vi "SSC DAQmx Disable Start Trigger.vi"(0 "DAQmx SSC in":T1[](array[typedef]), 11 "error in":errorcluster) -> (4 "DAQmx SSC out":T1[](array[typedef]), 15 "error out":errorcluster)   [LabVIEW 2020]
doc: "Configures the task to start acquiring or generating samples immediately upon starting the task."
uses:
  Pin Map/SSC DAQmx.ctl
  <vilib>/DAQmx/configure/trigger.llb/DAQmx Start Trigger (None).vi
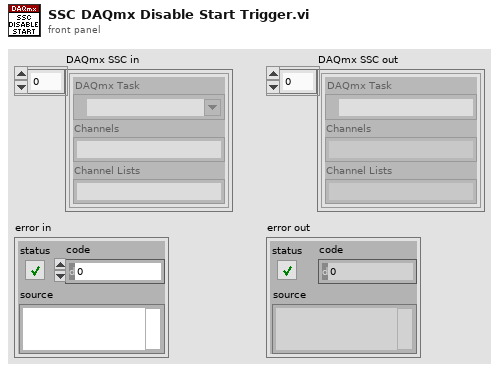
[diagram p1: front panel]
types:
  T1 = typedef "SSC DAQmx.ctl" = cluster{"DAQmx Task ":refnum<k21>, "Channels":string, "Channel Lists":string}
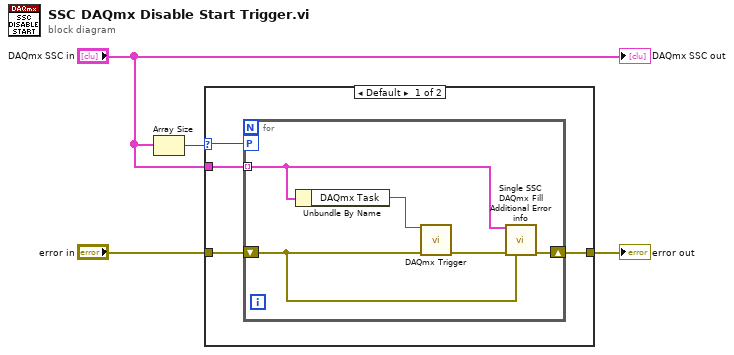
[diagram p0: block diagram]
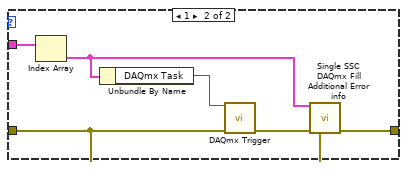
[diagram p2: hidden frame]
diagram:
  n1 = Array Size(array="DAQmx SSC in") -> (size(s)=w2:i32)
  n2 = case shown="Default" w2 {
    selector: w2 -> [w6 _]
    tunnel: [w8 w19] -> w4
    tunnel: "error in" -> [w7 w18]
    tunnel: "DAQmx SSC in" -> [w5 w17]
    frame Default {
      n3 = for {
        tunnel: w5 -> [w12] mode=indexing
        workers-P: w6 -> [_]
        shift-right: [w13] -> w8
        shift-left: w7 -> [w11]
        n4 = Unbundle By Name(w12) -> ("DAQmx Task"=w9:refnum<k21>)
        n5 = call-poly <vilib>:"DAQmx Trigger.vi"("task/channels in"=w9, "error in"=w11) -> ("error out"=w10:errorcluster)  [unwired: 12 in, 1 out]
        n6 = call "Single SSC DAQmx Fill Additional Error info.vi"("DAQmx SSC in"=w12, "error in"=w10, "previous error in"=w11) -> ("error out"=w13:errorcluster)  [unwired: 12 in]
      }
    }
    frame 1 {
      n7 = Index Array(array=w17) -> (element=w14:T1)  [unwired: 1 in]
      n8 = Unbundle By Name(w14) -> ("DAQmx Task"=w15:refnum<k21>)
      n9 = call-poly <vilib>:"DAQmx Trigger.vi"("task/channels in"=w15, "error in"=w18) -> ("error out"=w16:errorcluster)  [unwired: 12 in, 1 out]
      n10 = call "Single SSC DAQmx Fill Additional Error info.vi"("DAQmx SSC in"=w14, "error in"=w16, "previous error in"=w18) -> ("error out"=w19:errorcluster)  [unwired: 12 in]
    }
  }
  "error out" <- w4
  "DAQmx SSC out" <- "DAQmx SSC in"
